vi "PH_PSDBWriter.Wrap Waveform Data.vi"(0 "Name Array":string[](array[string]), 1 "Data Array":waveform(dbl)[](array[waveform]), 2 "x axis label Array":string[](array[string]), 3 "y axis label Array":string[](array[string]), 4 "x axis unit Array":string[](array[string]), 5 "y axis unit Array":string[](array[string]), 6 "Name Prefix":string) -> (17 "PSDB 2D Data Array":T1[](array[typedef]))   [LabVIEW 2014, in "PH_PSDBWriter.lvlib"]
doc: "This VI wrapes waveform data for the PSDB."
uses:
  PH_PSDBWriter.lvlib
  PH_PSDBWriter.2D dataset.ctl
  CSlibraries-extern/psdb_lv/PSDB_AxisDescription.ctl
  CSlibraries-extern/psdb_lv/PSDB.lvlib
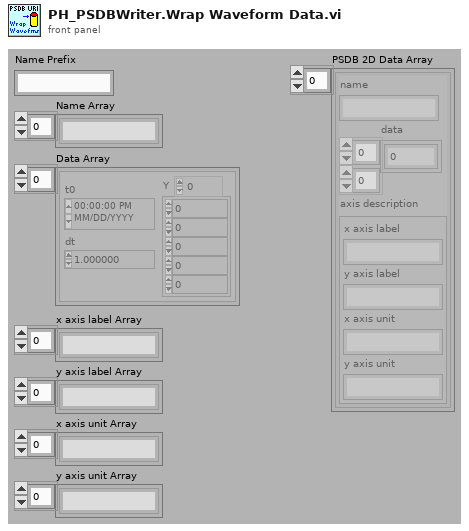
[diagram p1: front panel]
types:
  T1 = typedef "PH_PSDBWriter.lvlib/PH_PSDBWriter.2D dataset.ctl" = cluster{"name":string, "data":dbl[][], "axis description":T2}
  T2 = typedef "PSDB.lvlib/PSDB_AxisDescription.ctl" = cluster{"x axis label":string, "y axis label":string, "x axis unit":string, "y axis unit":string}
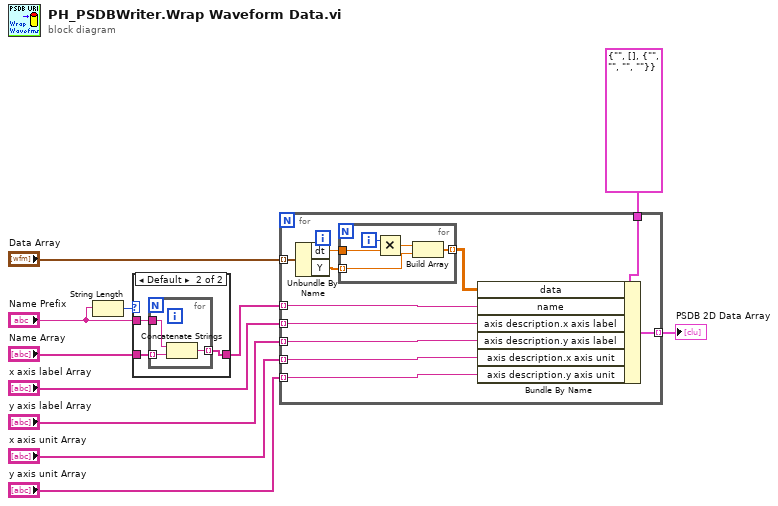
[diagram p0: block diagram]
diagram:
  n1 = String Length(string="Name Prefix") -> (length=w4:i32)
  n2 = case shown="Default" w4 {
    tunnel: "Name Array" -> [w12 w15]
    tunnel: [w12 w13] -> w1
    tunnel: "Name Prefix" -> [_ w14]
    frame 0 {
    }
    frame Default {
      n3 = for {
        tunnel: w15 -> [w18] mode=indexing
        tunnel: w14 -> [w17]
        tunnel: [w16] -> w13 mode=indexing
        n4 = Concatenate Strings(w17, w18) -> (w16:string)
      }
    }
  }
  n5 = for {
    tunnel: T1 {"name"="", "data"=[], "axis description"={"x axis label"="", "y axis label"="", "x axis unit"="", "y axis unit"=""}} ("2D data") -> [w29]
    tunnel: [w28] -> w9 mode=indexing
    tunnel: "Data Array" -> [w24] mode=indexing
    tunnel: w1 -> [w23] mode=indexing
    tunnel: "x axis label Array" -> [w22] mode=indexing
    tunnel: "y axis label Array" -> [w21] mode=indexing
    tunnel: "x axis unit Array" -> [w20] mode=indexing
    tunnel: "y axis unit Array" -> [w19] mode=indexing
    n6 = Unbundle By Name(w24) -> ("dt"=w27:dbl, "Y"=w26:dbl[])
    n7 = for {
      tunnel: w26 -> [w34] mode=indexing
      tunnel: w27 -> [w32]
      tunnel: [w30] -> w25 mode=indexing
      i -> [w33]
      n8 = Multiply(x=w33, y=w32) -> (x*y=w31:dbl)
      n9 = Build Array(w31, w34) -> (w30:dbl[])
    }
    n10 = Bundle By Name(cluster=w29, "data"=w25, "name"=w23, "axis description.x axis label"=w22, "axis description.y axis label"=w21, "axis description.x axis unit"=w20, "axis description.y axis unit"=w19) -> (w28:T1)
  }
  "PSDB 2D Data Array" <- w9
